vi "Open Audio.vi"(6 "Chunksize":i32, 8 "error in":errorcluster, 9 "Channels":i32, 10 "Format":u16 format="%.0x", 11 "Frequency":i32) -> (0 "error out":errorcluster, 3 "return":i32)   [LabVIEW 2015, in "LibSDL2_Mixer.lvlib"]
uses:
  LibSDL2_Mixer.lvlib
  LibSDL2 Wrapper/DLL/SDL2_mixer.dll
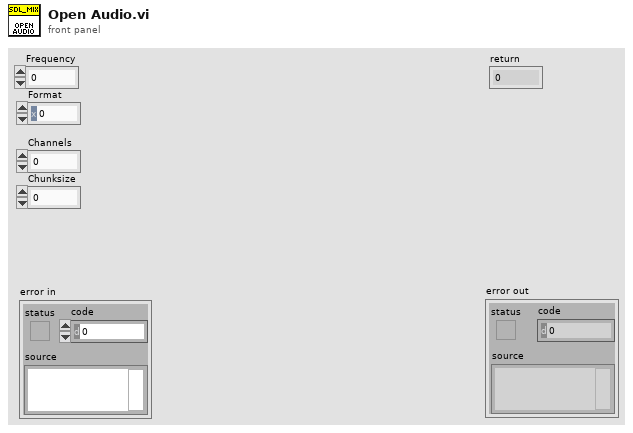
[diagram p1: front panel]
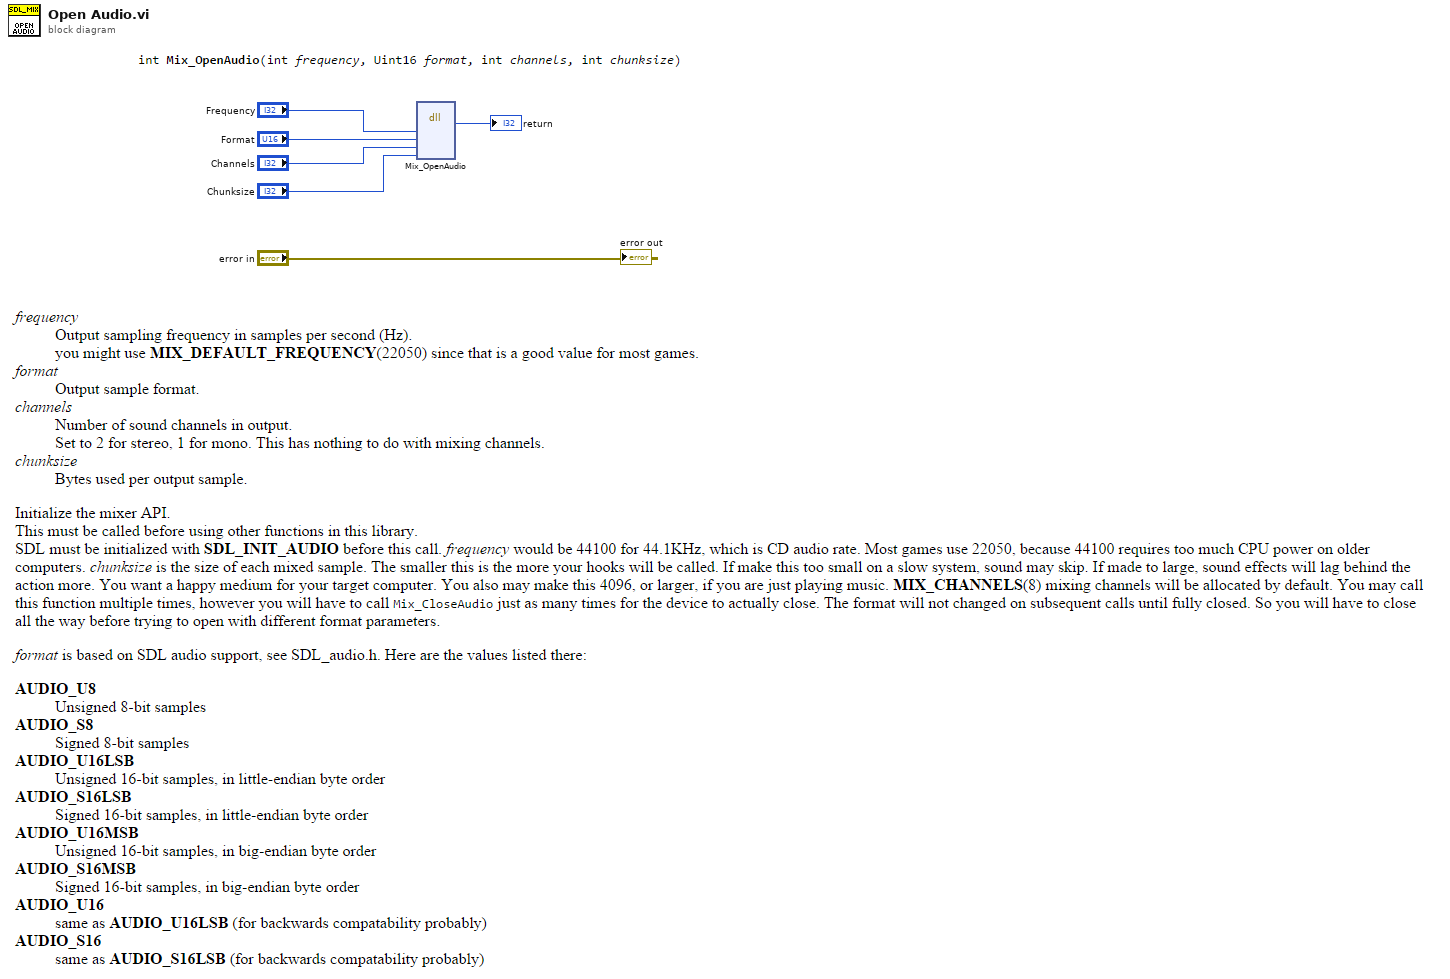
[diagram p0: block diagram]
diagram:
  n1 = dll-call lib="C:/dev/PGS/LabSDL2/Source/Libraries/LibSDL2 Wrapper/DLL/SDL2_mixer.dll" fn="Mix_OpenAudio"("frequency"="Frequency", "format"="Format", "channels"="Channels", "chunksize"="Chunksize") -> ("return type"=→"return":i32)  [unwired: 7 in, 2 out]
  "error out" <- "error in"
